vi "Get VI FP Reference.vi"(8 "error in (no error)":errorcluster, 11 "VI in":refnum<vi>) -> (0 "error out":errorcluster, 2 "Front Panel":refnum<vi>, 3 "VI out":refnum<vi>)   [LabVIEW 2019, in "VI Scripting Utilities.lvlib"]
uses:
  VI Scripting Utilities.lvlib
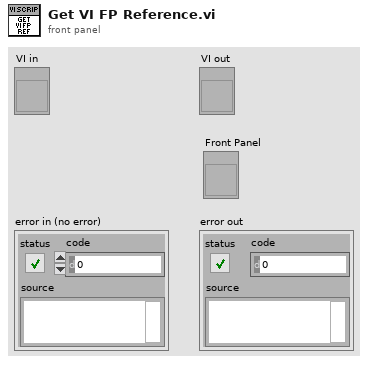
[diagram p1: front panel]
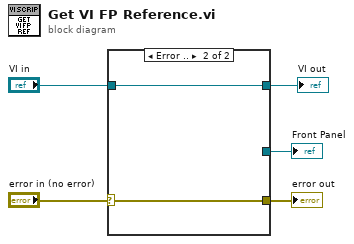
[diagram p0: block diagram]
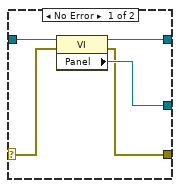
[diagram p2: hidden frame]
diagram:
  n1 = case shown="Error .." "error in (no error)" {
    selector: "error in (no error)" -> [w7 w12]
    tunnel: "VI in" -> [w10 w11]
    tunnel: [w9 w11] -> w4
    tunnel: [w8 _] -> w3
    tunnel: [w6 w12] -> w1
    frame No Error {
      n2 = property class="VI"(reference=w10, error in=w7) -> (reference out=w9:refnum<vi>, error out=w6:errorcluster, "Panel"=w8:refnum<vi>)
    }
    frame Error {
    }
  }
  "error out" <- w1
  "VI out" <- w4
  "Front Panel" <- w3
